vi "PIDDriveLooped.vi"() -> ()   [LabVIEW 2016]
uses:
  <vilib>/Rock Robotics/WPI/Utilities/WPI_GetSetVariantRefNum.vi
  <vilib>/addons/control/pid/pid.llb/PID (DBL).vi
  <vilib>/addons/control/pid/NI_PID_pid.lvlib
panel:
  in  "Finished PID":bool
  in  "Send":bool
  in  "Amount of Time (s)":dbl=7.0 format="%#_13g"
  out "Verify Graph":cluster{"X":dbl, "Y":dbl}[](graph)=[{"X"=0.0, "Y"=0.0}, {"X"=0.002403834311457255, "Y"=0.41939849398766105}, {"X"=0.009592158448876828, "Y"=0.8359196178093844}, {"X"=0.021530204216830304, "Y"=1.24957688435348}, {"X"=0.03818320341988926, "Y"=1.6603838065082581}, {"X"=0.05951638786262529, "Y"=2.0683538971620288}, {"X"=0.08549498934960995, "Y"=2.473500669203102}, {"X"=0.11608423968541483, "Y"=2.8758376355197877}, {"X"=0.15124937067461156, "Y"=3.2753783090003963}, {"X"=0.1909556141217717, "Y"=3.6721362025332374}, {"X"=0.23516820183146672, "Y"=4.066124829006621}, {"X"=0.2838523656082683, "Y"=4.457357701308857}, {"X"=0.3369733372567481, "Y"=4.8458483323282575}, {"X"=0.39449634858147764, "Y"=5.231610234953131}, {"X"=0.45638663138702834, "Y"=5.614656922071786}, {"X"=0.5226094174779721, "Y"=5.995001906572534}, {"X"=0.5931299386588802, "Y"=6.372658701343687}, {"X"=0.6679134267343245, "Y"=6.747640819273552}, {"X"=0.7469251135088762, "Y"=7.11996177325044}, {"X"=0.8301302307871071, "Y"=7.489635076162661}, {"X"=0.917494010373589, "Y"=7.856674240898527}, {"X"=1.0089816840728933, "Y"=8.221092780346344}, {"X"=1.1045584836895912, "Y"=8.582904207394426}, {"X"=1.204189641028255, "Y"=8.942122034931081}, {"X"=1.307840387893456, "Y"=9.298759775844621}, {"X"=1.4154759560897654, "Y"=9.652830943023353}, {"X"=1.5270615774217553, "Y"=10.004349049355591}, {"X"=1.6425624836939967, "Y"=10.35332760772964}, {"X"=1.761943906711062, "Y"=10.699780131033815}, {"X"=1.8851710782775222, "Y"=11.043720132156423}, {"X"=2.012209230197948, "Y"=11.385161123985775}, {"X"=2.1430235942769134, "Y"=11.72411661941018}, {"X"=2.2775794023189886, "Y"=12.060600131317951}, {"X"=2.4158418861287445, "Y"=12.394625172597397}, {"X"=2.5577762775107535, "Y"=12.726205256136824}, {"X"=2.703347808269587, "Y"=13.055353894824547}, {"X"=2.852521710209817, "Y"=13.382084601548875}, {"X"=3.0052632151360132, "Y"=13.706410889198114}, {"X"=3.1615375548527505, "Y"=14.028346270660581}, {"X"=3.3213099611645984, "Y"=14.347904258824581}, {"X"=3.4845456658761282, "Y"=14.665098366578427}, {"X"=3.651209900791912, "Y"=14.979942106810427}, {"X"=3.8212678977165218, "Y"=15.292448992408891}, {"X"=3.994684888454529, "Y"=15.60263253626213}, {"X"=4.171426104810503, "Y"=15.910506251258454}, {"X"=4.351456778589019, "Y"=16.216083650286173}, {"X"=4.534742141594647, "Y"=16.519378246233597}, {"X"=4.721247425631958, "Y"=16.820403551989035}, {"X"=4.910937862505524, "Y"=17.1191730804408}, {"X"=5.103778684019918, "Y"=17.415700344477198}, {"X"=5.29973512197971, "Y"=17.70999885698654}, {"X"=5.49877240818947, "Y"=18.00208213085714}, {"X"=5.700855774453773, "Y"=18.291963678977307}, {"X"=5.905950452577187, "Y"=18.579657014235345}, {"X"=6.114021674364287, "Y"=18.86517564951957}, {"X"=6.325034671619644, "Y"=19.148533097718293}, {"X"=6.538954676147828, "Y"=19.429742871719817}, {"X"=6.755746919753412, "Y"=19.708818484412458}, {"X"=6.975376634240967, "Y"=19.985773448684526}, {"X"=7.197809051415063, "Y"=20.26062127742433}, {"X"=7.423009403080272, "Y"=20.533375483520178}, {"X"=7.650942921041169, "Y"=20.804049579860383}, {"X"=7.881574837102323, "Y"=21.072657079333254}, {"X"=8.114870383068304, "Y"=21.3392114948271}, {"X"=8.350794790743688, "Y"=21.60372633923023}, {"X"=8.589313291933044, "Y"=21.866215125430962}, {"X"=8.830391118440943, "Y"=22.126691366317594}, {"X"=9.073993502071957, "Y"=22.385168574778447}, {"X"=9.320085674630658, "Y"=22.641660263701823}, {"X"=9.568632867921615, "Y"=22.896179945976034}, {"X"=9.819600313749405, "Y"=23.148741134489395}, {"X"=10.072953243918592, "Y"=23.399357342130212}, {"X"=10.328656890233757, "Y"=23.648042081786798}, {"X"=10.586676484499463, "Y"=23.894808866347457}, {"X"=10.846977258520285, "Y"=24.1396712087005}, {"X"=11.109524444100801, "Y"=24.382642621734245}, {"X"=11.37428327304557, "Y"=24.62373661833699}, {"X"=11.641218977159173, "Y"=24.86296671139706}, {"X"=11.910296788246178, "Y"=25.10034641380275}, {"X"=12.181481938111158, "Y"=25.335889238442384}, {"X"=12.454739658558681, "Y"=25.569608698204256}, {"X"=12.73003518139332, "Y"=25.801518305976685}, {"X"=13.007333738419652, "Y"=26.03163157464799}, {"X"=13.28660056144224, "Y"=26.259962017106464}, {"X"=13.567800882265669, "Y"=26.486523146240437}, {"X"=13.850899932694494, "Y"=26.711328474938195}, {"X"=14.135862944533296, "Y"=26.934391516088066}, {"X"=14.422655149586644, "Y"=27.155725782578354}, {"X"=14.71124177965911, "Y"=27.37534478729736}, {"X"=15.001588066555268, "Y"=27.593262043133414}, {"X"=15.293659242079684, "Y"=27.809491062974814}, {"X"=15.587420538036941, "Y"=28.024045359709874}, {"X"=15.882837186231594, "Y"=28.2369384462269}, {"X"=16.179874418468227, "Y"=28.448183835414202}, {"X"=16.478497466551406, "Y"=28.65779504016009}, {"X"=16.778671562285712, "Y"=28.86578557335288}, {"X"=17.0803619374757, "Y"=29.072168947880872}, {"X"=17.383533823925948, "Y"=29.27695867663239}, {"X"=17.68815245344104, "Y"=29.480168272495728}, {"X"=17.994183057825534, "Y"=29.68181124835921}, {"X"=18.301590868884006, "Y"=29.881901117111138}, {"X"=18.610341118421022, "Y"=30.080451391639823}, {"X"=18.920399038241168, "Y"=30.277475584833578}, {"X"=19.231729860149, "Y"=30.472987209580708}, {"X"=19.544298815949094, "Y"=30.666999778769537}, {"X"=19.85807113744602, "Y"=30.85952680528835}, {"X"=20.17301205644436, "Y"=31.050581802025476}, {"X"=20.48908680474868, "Y"=31.240178281869227}, {"X"=20.806260614163545, "Y"=31.4283297577079}, {"X"=21.124498716493537, "Y"=31.615049742429814}, {"X"=21.443766343543214, "Y"=31.80035174892328}, {"X"=21.76402872711716, "Y"=31.9842492900766}, {"X"=22.085251099019942, "Y"=32.16675587877809}, {"X"=22.40739869105613, "Y"=32.34788502791606}, {"X"=22.730436735030306, "Y"=32.52765025037882}, {"X"=23.054330462747025, "Y"=32.70606505905467}, {"X"=23.379045106010867, "Y"=32.88314296683194}, {"X"=23.704545896626406, "Y"=33.05889748659892}, {"X"=24.030798066398216, "Y"=33.23334213124394}, {"X"=24.35776684713085, "Y"=33.4064904136553}, {"X"=24.685417470628895, "Y"=33.578355846721294}, {"X"=25.01371516869693, "Y"=33.74895194333026}, {"X"=25.342625173139517, "Y"=33.918292216370496}, {"X"=25.672112715761223, "Y"=34.086390178730305}, {"X"=26.002143028366618, "Y"=34.253259343298005}, {"X"=26.332681342760296, "Y"=34.418913222961905}, {"X"=26.6636928907468, "Y"=34.58336533061032}, {"X"=26.995142904130716, "Y"=34.746629179131546}, {"X"=27.326996614716613, "Y"=34.908718281413904}, {"X"=27.659219254309065, "Y"=35.06964615034571}, {"X"=27.99177605471265, "Y"=35.229426298815255}, {"X"=28.32463224773192, "Y"=35.388072239710866}, {"X"=28.657753065171462, "Y"=35.54559748592085}, {"X"=28.99110373883584, "Y"=35.702015550333506}, {"X"=29.32464950052963, "Y"=35.857339945837154}, {"X"=29.658355582057403, "Y"=36.0115841853201}, {"X"=29.99218721522374, "Y"=36.16476178167067}, {"X"=30.32610963183319, "Y"=36.31688624777715}, {"X"=30.660088063690345, "Y"=36.46797109652786}, {"X"=30.994087742599767, "Y"=36.61802984081111}, {"X"=31.328073900366025, "Y"=36.76707599351521}, {"X"=31.662011768793697, "Y"=36.915123067528484}, {"X"=31.995866579687355, "Y"=37.06218457573921}, {"X"=32.32960356485157, "Y"=37.20827403103572}, {"X"=32.66318795609092, "Y"=37.353404946306334}, {"X"=32.99658498520996, "Y"=37.497590834439336}, {"X"=33.329759884013264, "Y"=37.64084520832305}, {"X"=33.66267788430541, "Y"=37.78318158084579}, {"X"=33.99530421789097, "Y"=37.92461346489586}, {"X"=34.327604116574534, "Y"=38.06515437336158}, {"X"=34.65954281216064, "Y"=38.20481781913123}, {"X"=34.991085536453866, "Y"=38.34361731509315}, {"X"=35.32219752125879, "Y"=38.481566374135646}, {"X"=35.65284399838, "Y"=38.618678509147024}, {"X"=35.98299019962205, "Y"=38.754967233015584}, {"X"=36.31260135678951, "Y"=38.89044605862966}, {"X"=36.64164270168696, "Y"=39.025128498877535}, {"X"=36.97007946611896, "Y"=39.15902806664754}, {"X"=37.2978768818901, "Y"=39.29215827482796}, {"X"=37.62500018080493, "Y"=39.424532636307134}, {"X"=37.95141459466804, "Y"=39.55616466397336}, {"X"=38.27708535528399, "Y"=39.68706787071495}, {"X"=38.601977694457354, "Y"=39.81725576942021}, {"X"=38.92605684399272, "Y"=39.946741872977455}, {"X"=39.249288035694626, "Y"=40.07553969427498}, {"X"=39.57163650136766, "Y"=40.203662746201125}, {"X"=39.893067472816405, "Y"=40.331124541644165}, {"X"=40.21354618184543, "Y"=40.45793859349244}, {"X"=40.53303786025929, "Y"=40.58411841463423}, {"X"=40.85150773986257, "Y"=40.70967751795787}, {"X"=41.16892105245982, "Y"=40.834629416351675}, {"X"=41.48524302985565, "Y"=40.95898762270393}, {"X"=41.80043890385462, "Y"=41.08276564990297}, {"X"=42.11447390626127, "Y"=41.205977010837074}, {"X"=42.427313268880205, "Y"=41.328635218394574}, {"X"=42.738922223515985, "Y"=41.45075378546379}, {"X"=43.04926600197319, "Y"=41.57234622493301}, {"X"=43.35830983605638, "Y"=41.69342604969056}, {"X"=43.666018957570124, "Y"=41.81400677262473}, {"X"=43.972358598319005, "Y"=41.934101906623845}, {"X"=44.27729399010758, "Y"=42.053724964576226}, {"X"=44.58079036474045, "Y"=42.172889459370154}, {"X"=44.882812954022164, "Y"=42.29160890389396}, {"X"=45.18332698975728, "Y"=42.40989681103595}, {"X"=45.48229770375039, "Y"=42.527766693684434}, {"X"=45.77969032780607, "Y"=42.64523206472772}, {"X"=46.07547009372889, "Y"=42.76230643705412}, {"X"=46.369602233323405, "Y"=42.87900332355195}, {"X"=46.662051978394196, "Y"=42.995336237109505}, {"X"=46.952784560745826, "Y"=43.11131869061511}, {"X"=47.2417652121829, "Y"=43.22696419695706}, {"X"=47.52895916450995, "Y"=43.34228626902369}, {"X"=47.81433164953157, "Y"=43.45729841970327}, {"X"=48.09784789905231, "Y"=43.57201416188414}, {"X"=48.37947314487676, "Y"=43.686447008454614}, {"X"=48.6591726188095, "Y"=43.80061047230299}, {"X"=48.93691155265508, "Y"=43.914518066317584}, {"X"=49.212655178218085, "Y"=44.02818330338668}, {"X"=49.48636872730308, "Y"=44.14161969639863}, {"X"=49.75801743171465, "Y"=44.25484075824171}, {"X"=50.027566523257335, "Y"=44.36786000180426}, {"X"=50.29498123373574, "Y"=44.48069093997457}, {"X"=50.56022679495441, "Y"=44.59334708564095}, {"X"=50.823268438717946, "Y"=44.70584195169171}, {"X"=51.08407139683091, "Y"=44.818189051015175}, {"X"=51.34260090109785, "Y"=44.93040189649964}, {"X"=51.59882218332336, "Y"=45.04249400103342}, {"X"=51.852700475312005, "Y"=45.154478877504815}, {"X"=52.10420100886837, "Y"=45.26637003880216}, {"X"=52.353289015797, "Y"=45.378180997813736}, {"X"=52.59992972790249, "Y"=45.48992526742788}, {"X"=52.8440883769894, "Y"=45.60161636053288}, {"X"=53.08573019486229, "Y"=45.713267790017056}, {"X"=53.32482041332578, "Y"=45.824893068768716}, {"X"=53.561324264184385, "Y"=45.93650570967617}, {"X"=53.7952069792427, "Y"=46.04811922562773}, {"X"=54.0264337903053, "Y"=46.159747129511715}, {"X"=54.25496992917675, "Y"=46.27140293421641}, {"X"=54.48078062766162, "Y"=46.38310015263014}, {"X"=54.7038311175645, "Y"=46.49485229764122}, {"X"=54.92408663068993, "Y"=46.606672882137964}, {"X"=55.14151239884251, "Y"=46.71857541900866}, {"X"=55.356073653826805, "Y"=46.830573421141644}, {"X"=55.56773562744737, "Y"=46.9426804014252}, {"X"=55.77646355150879, "Y"=47.05490987274766}, {"X"=55.98222265781563, "Y"=47.167275347997325}, {"X"=56.18497817817248, "Y"=47.279790340062505}, {"X"=56.3846953443839, "Y"=47.39246836183151}, {"X"=56.58133938825444, "Y"=47.50532292619265}, {"X"=56.77487554158871, "Y"=47.61836754603424}, {"X"=56.96526903619125, "Y"=47.731615734244585}, {"X"=57.15248510386666, "Y"=47.845081003712}, {"X"=57.33648897641948, "Y"=47.95877686732478}, {"X"=57.51724588565432, "Y"=48.07271683797124}, {"X"=57.69472106337571, "Y"=48.186914428539716}, {"X"=57.868879741388234, "Y"=48.30138315191849}, {"X"=58.03968715149649, "Y"=48.416136520995884}, {"X"=58.20710852550503, "Y"=48.5311880486602}, {"X"=58.37110909521841, "Y"=48.64655124779974}, {"X"=58.53165409244122, "Y"=48.76223963130285}, {"X"=58.68870874897804, "Y"=48.8782667120578}, {"X"=58.84223829663342, "Y"=48.994646002952926}, {"X"=58.99220796721195, "Y"=49.11139101687652}, {"X"=59.138582992518195, "Y"=49.2285152667169}, {"X"=59.28132860435671, "Y"=49.34603226536239}, {"X"=59.4204100345321, "Y"=49.46395552570128}, {"X"=59.55579251484891, "Y"=49.58229856062189}, {"X"=59.68744127711172, "Y"=49.70107488301252}, {"X"=59.8153215531251, "Y"=49.82029800576148}, {"X"=59.93939857469362, "Y"=49.9399814417571}, {"X"=60.05963857964622, "Y"=50.060138261910026}, {"X"=60.176030944371796, "Y"=50.18077137164493}, {"X"=60.2885881838193, "Y"=50.30187351090052}, {"X"=60.397323818962015, "Y"=50.42343697763785}, {"X"=60.50225137077323, "Y"=50.545454069817964}, {"X"=60.60338436022622, "Y"=50.6679170854019}, {"X"=60.70073630829428, "Y"=50.790818322350724}, {"X"=60.794320735950684, "Y"=50.914150078625475}, {"X"=60.88415116416872, "Y"=51.03790465218721}, {"X"=60.97024111392168, "Y"=51.16207434099697}, {"X"=61.052604106182834, "Y"=51.286651443015806}, {"X"=61.13125366192548, "Y"=51.411628256204764}, {"X"=61.20620330212289, "Y"=51.5369970785249}, {"X"=61.27746654774836, "Y"=51.66275020793726}, {"X"=61.34505691977516, "Y"=51.788879942402886}, {"X"=61.40898793917659, "Y"=51.91537857988284}, {"X"=61.46927312692593, "Y"=52.04223841833816}, {"X"=61.52592600399646, "Y"=52.169451755729895}, {"X"=61.578960091361466, "Y"=52.2970108900191}, {"X"=61.628388909994236, "Y"=52.42490811916683}, {"X"=61.674225980868044, "Y"=52.55313574113411}, {"X"=61.71648482495618, "Y"=52.68168605388202}, {"X"=61.75517896323194, "Y"=52.81055135537158}, {"X"=61.79032191666859, "Y"=52.93972394356386}, {"X"=61.82192720623943, "Y"=53.069196116419896}, {"X"=61.850008352917726, "Y"=53.198960171900744}, {"X"=61.87457887767678, "Y"=53.32900840796744}, {"X"=61.89565230148987, "Y"=53.459333122581064}, {"X"=61.91324214533027, "Y"=53.58992661370263}, {"X"=61.92736193017129, "Y"=53.720781179293205}, {"X"=61.93802517698619, "Y"=53.85188911731383}, {"X"=61.945245406748256, "Y"=53.98324272572556}, {"X"=61.94903614043079, "Y"=54.11483430248945}, {"X"=61.94941089900706, "Y"=54.24665614556653}, {"X"=61.94638320345036, "Y"=54.37870055291786}, {"X"=61.939966574733965, "Y"=54.51095982250449}, {"X"=61.93017453383116, "Y"=54.64342625228747}, {"X"=61.917020601715244, "Y"=54.776092140227846}, {"X"=61.90051829935948, "Y"=54.90894978428667}, {"X"=61.88068114773718, "Y"=55.041991482424976}, {"X"=61.8575226678216, "Y"=55.17520953260384}, {"X"=61.831056380586034, "Y"=55.30859623278428}, {"X"=61.801295807003775, "Y"=55.44214388092737}, {"X"=61.7682544680481, "Y"=55.57584477499415}, {"X"=61.73194588469229, "Y"=55.709691212945664}, {"X"=61.69238357790963, "Y"=55.84367549274297}, {"X"=61.64958106867341, "Y"=55.977789912347106}, {"X"=61.60355187795692, "Y"=56.11202676971913}, {"X"=61.554309526733434, "Y"=56.24637836282009}, {"X"=61.50186753597624, "Y"=56.380836989611026}, {"X"=61.446239426658614, "Y"=56.515394948053}, {"X"=61.38743871975385, "Y"=56.650044536107046}, {"X"=61.32547893623523, "Y"=56.784778051734236}, {"X"=61.26037359707603, "Y"=56.9195877928956}, {"X"=61.192136223249555, "Y"=57.054466057552176}, {"X"=61.12078033572907, "Y"=57.18940514366504}, {"X"=61.046319455487875, "Y"=57.32439734919522}, {"X"=60.96876710349924, "Y"=57.459434972103786}, {"X"=60.88813680073645, "Y"=57.59451031035177}, {"X"=60.8044420681728, "Y"=57.729615661900226}, {"X"=60.717696426781565, "Y"=57.864743324710204}, {"X"=60.627913397536034, "Y"=57.99988559674275}, {"X"=60.53510650140949, "Y"=58.13503477595891}, {"X"=60.439289259375215, "Y"=58.27018316031974}, {"X"=60.3404751924065, "Y"=58.40532304778628}, {"X"=60.23867782147662, "Y"=58.540446736319595}, {"X"=60.133910667558865, "Y"=58.67554652388072}, {"X"=60.026187251626524, "Y"=58.8106147084307}, {"X"=59.915521094652874, "Y"=58.9456435879306}, {"X"=59.801925717611205, "Y"=59.08062546034145}, {"X"=59.68541464147479, "Y"=59.21555262362432}, {"X"=59.56600138721692, "Y"=59.35041737574024}, {"X"=59.443699475810895, "Y"=59.48521201465027}, {"X"=59.31852242822997, "Y"=59.61992883831546}, {"X"=59.19048376544745, "Y"=59.754560144696846}, {"X"=59.05959700843661, "Y"=59.8890982317555}, {"X"=58.92587567817074, "Y"=60.02353539745244}, {"X"=58.78933329562313, "Y"=60.15786393974874}, {"X"=58.64998338176704, "Y"=60.29207615660544}, {"X"=58.50783945757579, "Y"=60.42616434598358}, {"X"=58.36291504402263, "Y"=60.56012080584423}, {"X"=58.21522366208086, "Y"=60.69393783414842}, {"X"=58.064778832723775, "Y"=60.8276077288572}, {"X"=57.91159407692464, "Y"=60.96112278793164}, {"X"=57.75568291565674, "Y"=61.094475309332765}, {"X"=57.59705886989338, "Y"=61.227657591021625}, {"X"=57.43573546060783, "Y"=61.36066193095929}, {"X"=57.27172620877337, "Y"=61.493480627106784}, {"X"=57.10504463536329, "Y"=61.62610597742517}, {"X"=56.93570426135088, "Y"=61.7585302798755}, {"X"=56.763718607709414, "Y"=61.89074583241881}, {"X"=56.58910119541218, "Y"=62.022744933016156}, {"X"=56.41186554543247, "Y"=62.15451987962858}, {"X"=56.23202517874355, "Y"=62.28606297021715}, {"X"=56.04959361631872, "Y"=62.4173665027429}, {"X"=55.86458437913127, "Y"=62.54842277516687}, {"X"=55.67701098815446, "Y"=62.67922408545013}, {"X"=55.4868869643616, "Y"=62.80976273155371}, {"X"=55.294225828725956, "Y"=62.94003101143868}, {"X"=55.099041102220816, "Y"=63.07002122306607}, {"X"=54.90134630581948, "Y"=63.19972566439694}, {"X"=54.70115496049521, "Y"=63.329136633392324}, {"X"=54.498480587221316, "Y"=63.45824642801328}, {"X"=54.29333670697105, "Y"=63.58704734622087}, {"X"=54.085736840717715, "Y"=63.71553168597613}, {"X"=53.8756945094346, "Y"=63.8436917452401}, {"X"=53.66322323409498, "Y"=63.97151982197384}, {"X"=53.448336535672134, "Y"=64.09900821413841}, {"X"=53.23104793513937, "Y"=64.22614921969483}, {"X"=53.01137095346995, "Y"=64.35293513660417}, {"X"=52.78931911163717, "Y"=64.47935826282747}, {"X"=52.564905930614295, "Y"=64.60541089632581}, {"X"=52.33814493137463, "Y"=64.73108533506019}, {"X"=52.10904963489146, "Y"=64.85637387699168}, {"X"=51.87763356213806, "Y"=64.98126882008134}, {"X"=51.64391023408773, "Y"=65.10576246229019}, {"X"=51.40789317171371, "Y"=65.22984710157931}, {"X"=51.16959589598933, "Y"=65.35351503590974}, {"X"=50.92903192788787, "Y"=65.47675856324251}, {"X"=50.68621478838259, "Y"=65.59956998153869}, {"X"=50.44115799844681, "Y"=65.72194158875934}, {"X"=50.19387507905377, "Y"=65.84386568286547}, {"X"=49.94437955117677, "Y"=65.96533456181817}, {"X"=49.69268493578913, "Y"=66.08634052357844}, {"X"=49.43880475386409, "Y"=66.2068758661074}, {"X"=49.18275252637494, "Y"=66.32693288736603}, {"X"=48.924541774295, "Y"=66.4465038853154}, {"X"=48.66418601859751, "Y"=66.56558115791657}, {"X"=48.40169878025579, "Y"=66.6841570031306}, {"X"=48.13709358024309, "Y"=66.8022237189185}, {"X"=47.870383939532715, "Y"=66.91977360324137}, {"X"=47.60158337909796, "Y"=67.0367989540602}, {"X"=47.33070541991208, "Y"=67.15329206933609}, {"X"=47.05776358294839, "Y"=67.26924524703006}, {"X"=46.78277138918015, "Y"=67.38465078510316}, {"X"=46.50574235958064, "Y"=67.49950098151646}, {"X"=46.22669001512318, "Y"=67.61378813423099}, {"X"=45.94562787678102, "Y"=67.72750454120781}, {"X"=45.66256946552747, "Y"=67.84064250040795}, {"X"=45.37752830233579, "Y"=67.95319430979248}, {"X"=45.090517908179265, "Y"=68.06515226732245}, {"X"=44.80155180403122, "Y"=68.17650867095887}, {"X"=44.51064351086487, "Y"=68.28725581866284}, {"X"=44.217806549653574, "Y"=68.39738600839539}, {"X"=43.92305444137057, "Y"=68.50689153811756}, {"X"=43.62640070698913, "Y"=68.6157647057904}, {"X"=43.32785886748259, "Y"=68.72399780937496}, {"X"=43.027442443824185, "Y"=68.83158314683232}, {"X"=42.72516495698723, "Y"=68.93851301612347}, {"X"=42.42103992794502, "Y"=69.0447797152095}, {"X"=42.11508087767078, "Y"=69.15037554205145}, {"X"=41.807301327137864, "Y"=69.25529279461037}, {"X"=41.4977147973195, "Y"=69.3595237708473}, {"X"=41.186334809189006, "Y"=69.46306076872331}, {"X"=40.87317488371967, "Y"=69.56589608619943}, {"X"=40.558248541884744, "Y"=69.66802202123671}, {"X"=40.24156930465756, "Y"=69.7694308717962}, {"X"=39.92315069301135, "Y"=69.87011493583896}, {"X"=39.60300622791944, "Y"=69.97006651132602}, {"X"=39.28114943035509, "Y"=70.06927789621844}, {"X"=38.95759382129158, "Y"=70.16774138847728}, {"X"=38.632352921702235, "Y"=70.26544928606356}, {"X"=38.30544025256029, "Y"=70.36239388693835}, {"X"=37.97686933483905, "Y"=70.4585674890627}, {"X"=37.646653689511815, "Y"=70.55396239039766}, {"X"=37.31480683755183, "Y"=70.64857088890426}, {"X"=36.98134229993241, "Y"=70.74238528254357}, {"X"=36.646273597626845, "Y"=70.83539786927662}, {"X"=36.309614251608394, "Y"=70.92760094706448}, {"X"=35.971377782850375, "Y"=71.01898681386817}, {"X"=35.63157771232602, "Y"=71.10954776764878}, {"X"=35.290227561008656, "Y"=71.19927610636732}, {"X"=34.94734084987158, "Y"=71.28816412798486}, {"X"=34.602931099888025, "Y"=71.37620413046244}, {"X"=34.257011832031324, "Y"=71.46338841176112}, {"X"=33.909596567274704, "Y"=71.54970926984194}, {"X"=33.560698826591505, "Y"=71.63515900266594}, {"X"=33.21033213095501, "Y"=71.71972990819418}, {"X"=32.85851000133846, "Y"=71.80341428438771}, {"X"=32.50524595871519, "Y"=71.8862044292076}, {"X"=32.150553524058424, "Y"=71.96809264061484}, {"X"=31.794446218341495, "Y"=72.04907121657052}, {"X"=31.436937562537693, "Y"=72.1291324550357}, {"X"=31.07804107762026, "Y"=72.2082686539714}, {"X"=30.717770284562526, "Y"=72.2864721113387}, {"X"=30.356138704337727, "Y"=72.36373512509861}, {"X"=29.99315985791917, "Y"=72.4400499932122}, {"X"=29.628847266280175, "Y"=72.51540901364052}, {"X"=29.26321445039396, "Y"=72.58980448434463}, {"X"=28.896274931233847, "Y"=72.66322870328555}, {"X"=28.528042229773142, "Y"=72.73567396842435}, {"X"=28.158529866985077, "Y"=72.80713257772207}, {"X"=27.787751363842986, "Y"=72.87759682913976}, {"X"=27.41572024132011, "Y"=72.94705902063848}, {"X"=27.042450020389744, "Y"=73.01551145017926}, {"X"=26.66795422202521, "Y"=73.08294641572316}, {"X"=26.292246367199745, "Y"=73.14935621523124}, {"X"=25.915339976886678, "Y"=73.21473314666451}, {"X"=25.537248572059234, "Y"=73.27906950798408}, {"X"=25.15798567369074, "Y"=73.34235759715094}, {"X"=24.77756480275449, "Y"=73.40458971212617}, {"X"=24.395999480223722, "Y"=73.46575815087081}, {"X"=24.01330322707178, "Y"=73.52585521134591}, {"X"=23.629489564271893, "Y"=73.58487319151253}, {"X"=23.244572012797356, "Y"=73.6428043893317}, {"X"=22.85856409362151, "Y"=73.69964110276447}, {"X"=22.471479327717553, "Y"=73.7553756297719}, {"X"=22.083331236058854, "Y"=73.81000026831504}, {"X"=21.694133339618624, "Y"=73.86350731635494}, {"X"=21.30389915937016, "Y"=73.91588907185263}, {"X"=20.912642216286805, "Y"=73.96713783276918}, {"X"=20.520376031341776, "Y"=74.01724589706564}, {"X"=20.127114125508392, "Y"=74.06620556270303}, {"X"=19.732870019759957, "Y"=74.11400912764242}, {"X"=19.337657235069685, "Y"=74.16064888984488}, {"X"=18.941489292410935, "Y"=74.20611714727141}, {"X"=18.544379712756943, "Y"=74.2504061978831}, {"X"=18.146342017081004, "Y"=74.29350833964098}, {"X"=17.747389726356438, "Y"=74.3354158705061}, {"X"=17.34753636155647, "Y"=74.3761210884395}, {"X"=16.946795443654445, "Y"=74.41561629140226}, {"X"=16.545180493623583, "Y"=74.4538937773554}, {"X"=16.142705032437206, "Y"=74.49094584425998}, {"X"=15.739382581068632, "Y"=74.52676479007707}, {"X"=15.33522666049106, "Y"=74.56134291276766}, {"X"=14.93025079167785, "Y"=74.59467251029285}, {"X"=14.524468495602243, "Y"=74.62674588061368}, {"X"=14.117893293237543, "Y"=74.65755532169119}, {"X"=13.710538705557042, "Y"=74.68709313148642}, {"X"=13.302418253533986, "Y"=74.71535160796044}, {"X"=12.893545458141716, "Y"=74.74232304907429}, {"X"=12.483933840353458, "Y"=74.76799975278902}, {"X"=12.073596921142531, "Y"=74.79237401706567}, {"X"=11.662548221482247, "Y"=74.81543813986531}, {"X"=11.250801262345803, "Y"=74.83718441914895}, {"X"=10.83836956470656, "Y"=74.85760515287768}, {"X"=10.425266649537782, "Y"=74.87669263901253}, {"X"=10.011506037812751, "Y"=74.89443917551456}, {"X"=9.597101250504764, "Y"=74.9108370603448}, {"X"=9.182065808587055, "Y"=74.92587859146431}, {"X"=8.766413233032956, "Y"=74.93955606683414}, {"X"=8.35015704481576, "Y"=74.95186178441534}, {"X"=7.933310764908711, "Y"=74.96278804216897}, {"X"=7.515887914285145, "Y"=74.97232713805604}, {"X"=7.097902013918272, "Y"=74.98047137003763}, {"X"=6.679366584781441, "Y"=74.98721303607478}, {"X"=6.260295147847927, "Y"=74.99254443412855}, {"X"=5.840701224090978, "Y"=74.99645786215997}, {"X"=5.420598334483934, "Y"=74.99894561813011}, {"X"=5.000000000000007, "Y"=75.0}]
  in  "PID Segments (1-500)":dbl=150.0
  in  "Limit of Orientation Change":dbl=30.0
  in  "Absolute Theta Final":dbl=-1.57
  in  "Absolute Theta initial":dbl
  in  "Y":dbl[](array[numeric])=[0.0, 60.0, 5.0]
  in  "X":dbl[](array[numeric])=[0.0, 50.0, 75.0]
  out "throttle":dbl=-0.8 format="%.2f"
  out "steer":dbl=0.8 format="%.2f"
  out "Waveform Chart":cluster{dbl, "setpoint":dbl}(graph)={92.439765, "setpoint"=131.40149028791936}
  out "Waveform Chart 2":cluster{"Yaw Wind":dbl, "setpoint":dbl}(graph)={"Yaw Wind"=0.830122225479803, "setpoint"=1.5429574932445604}
  in  "Manual":bool
  in  "Steer Range":cluster{"output high":dbl, "output low":dbl}={"output high"=0.8, "output low"=-0.8} {"output low" format="%.2f"; "output high" format="%.2f"}
  in  "PID Steer gains":T1={"proportional gain (Kc)"=1.0, "integral time (Ti, min)"=0.01, "derivative time (Td, min)"=0.0} {"derivative time (Td, min)" format="%.3f"; "integral time (Ti, min)" format="%.3f"; "proportional gain (Kc)" format="%.3f"}
  in  "Speed Range":cluster{"output high":dbl, "output low":dbl}={"output high"=0.8, "output low"=-0.8} {"output low" format="%.2f"; "output high" format="%.2f"}
  in  "PID Speed gains":T1={"proportional gain (Kc)"=0.04, "integral time (Ti, min)"=0.0, "derivative time (Td, min)"=0.0} {"derivative time (Td, min)" format="%.3f"; "integral time (Ti, min)" format="%.3f"; "proportional gain (Kc)" format="%.3f"}
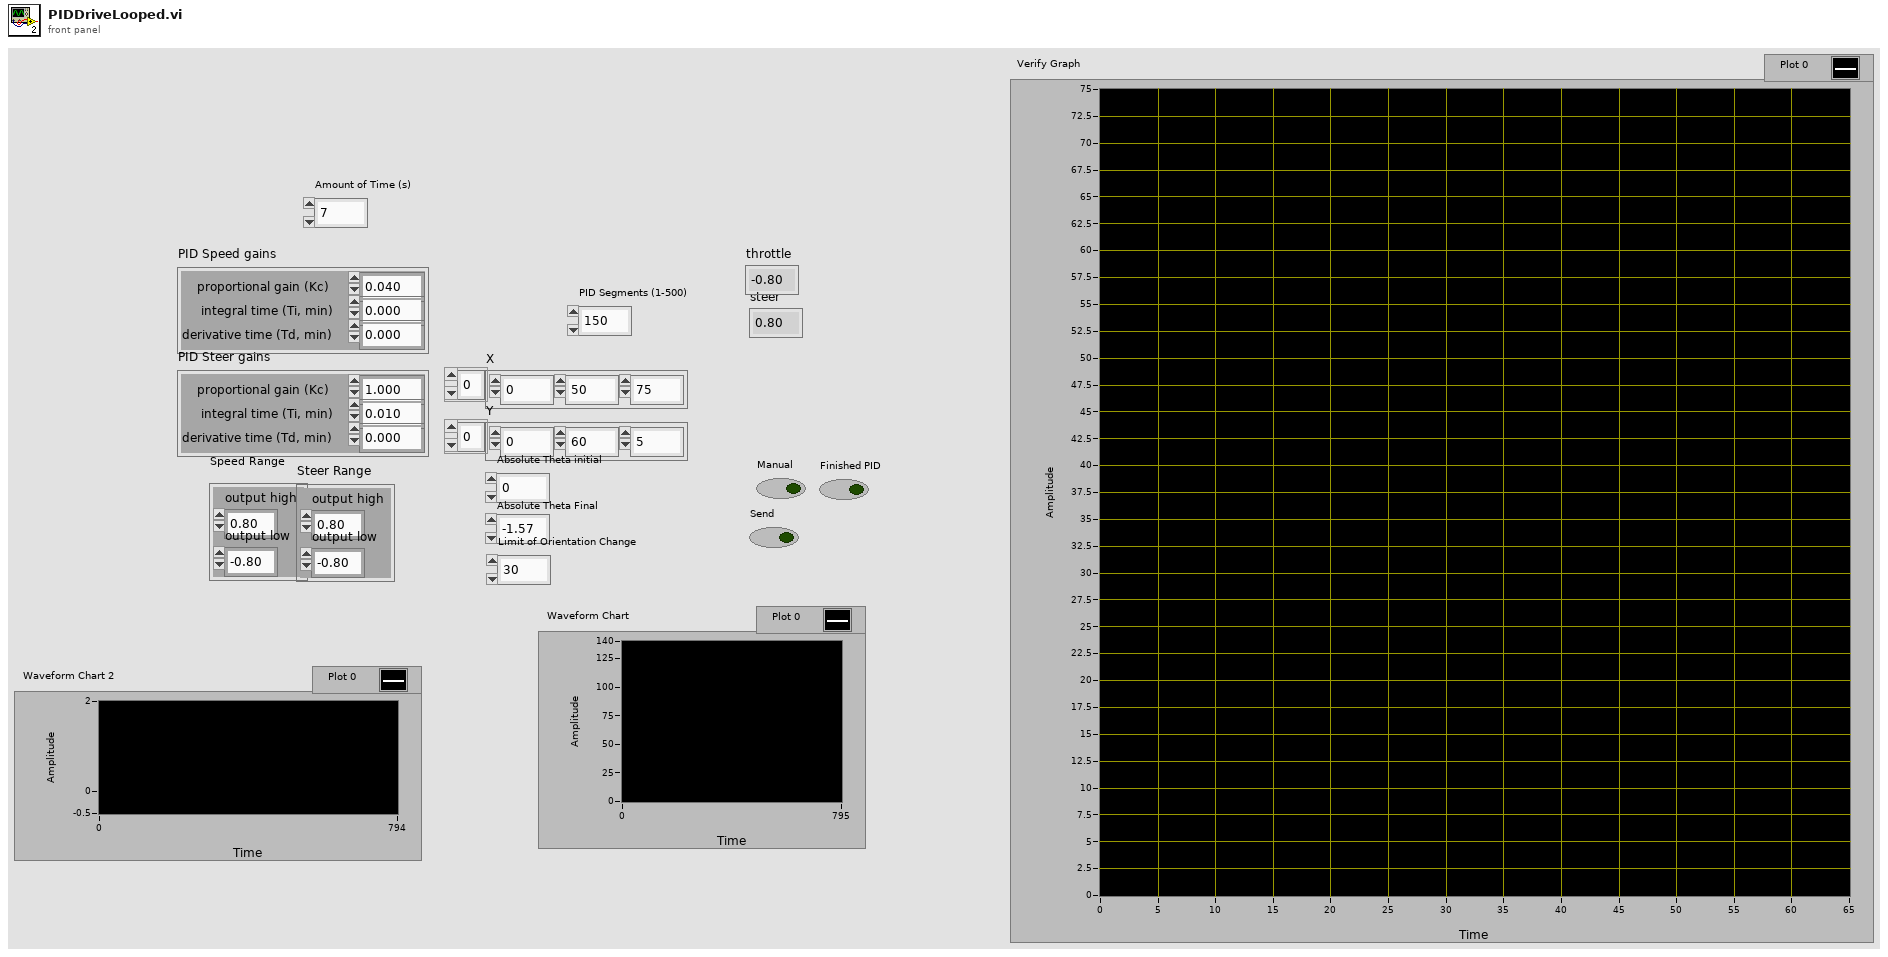
[diagram p1: front panel]
types:
  T1 = cluster{"proportional gain (Kc)":dbl, "integral time (Ti, min)":dbl, "derivative time (Td, min)":dbl}
  T2 = typedef "WPI_MotorControlDeviceRef.ctl" = cluster{"DeviceStatus":errorcluster, "Type":T3, "PWM":cluster{"PWM Channel":T4, "DeadBand":T5}, "CAN":cluster{"Device Number":u8, "SetOutput VI Ref":variant, "GetOutput VI Ref":variant, "Enable VI Ref":variant, "Disable VI Ref":variant, "Data":variant}, "Invert":bool}
  T3 = typedef "WPI_MotorControlType.ctl" = enum16{"PWM", "CAN"}
  T4 = typedef "FPGA_DIOPWMChannel.ctl" = enum8{"PWM 0", "PWM 1", "PWM 2", "PWM 3", "PWM 4", "PWM 5", "PWM 6", "PWM 7", "PWM 8", "PWM 9", "PWM MXP 0", "PWM MXP 1", "PWM MXP 2", "PWM MXP 3", "PWM MXP 4", "PWM MXP 5", "PWM MXP 6", "PWM MXP 7", "PWM MXP 8", "PWM MXP 9", "Invalid"}
  T5 = typedef "WPI_PWMDeadband.ctl" = cluster{"Name":string, "maxPositivePwm":i32, "minPositivePwm":i32, "centerPwm":i32, "maxNegativePwm":i32, "minNegativePwm":i32, "angularRange":u16}
  T6 = typedef "WPI_JoystickDevRef.ctl" = cluster{"Device":T7}
  T7 = typedef "WPI_JoystickDeviceEnum.ctl" = enum16{"USB 0", "USB 1", "USB 2", "USB 3", "USB 4", "USB 5"}
  T8 = typedef "WPI_EncoderDevRef.ctl" = cluster{"DevStatus":errorcluster, "EncoderIndex":T9, "CounterIndex":T10, "DistancePerCount":dbl, "Decoding Type":T11}
  T9 = typedef "FPGA_EncoderIdx.ctl" = enum8{"Enc 0", "Enc 1", "Enc 2", "Enc 3", "Enc 4", "Enc 5", "Enc 6", "Enc 7", "Invalid"}
  T10 = typedef "FPGA_CounterCtrSystemIndex.ctl" = enum8{"Ctr 0", "Ctr 1", "Ctr 2", "Ctr 3", "Ctr 4", "Ctr 5", "Ctr 6", "Ctr 7", "Invalid"}
  T11 = typedef "WPI_EncoderType.ctl" = enum16{"1x", "2x", "4x"}
  T12 = typedef "WPI_I2CDevRef.ctl" = cluster{"DevStatus":errorcluster, "Device Address":u8, "Handle":i32, "I2C Bus":T13}
  T13 = typedef "i2c_bus.ctl" = enum16{"I2C On-Board", "I2C MXP", "Invalid"}
  T14 = cluster{"Yaw":dbl, "Roll":dbl, "Pitch":dbl, "Yaw Wind":dbl, "Roll Wind":dbl, "Pitch Wind":dbl}
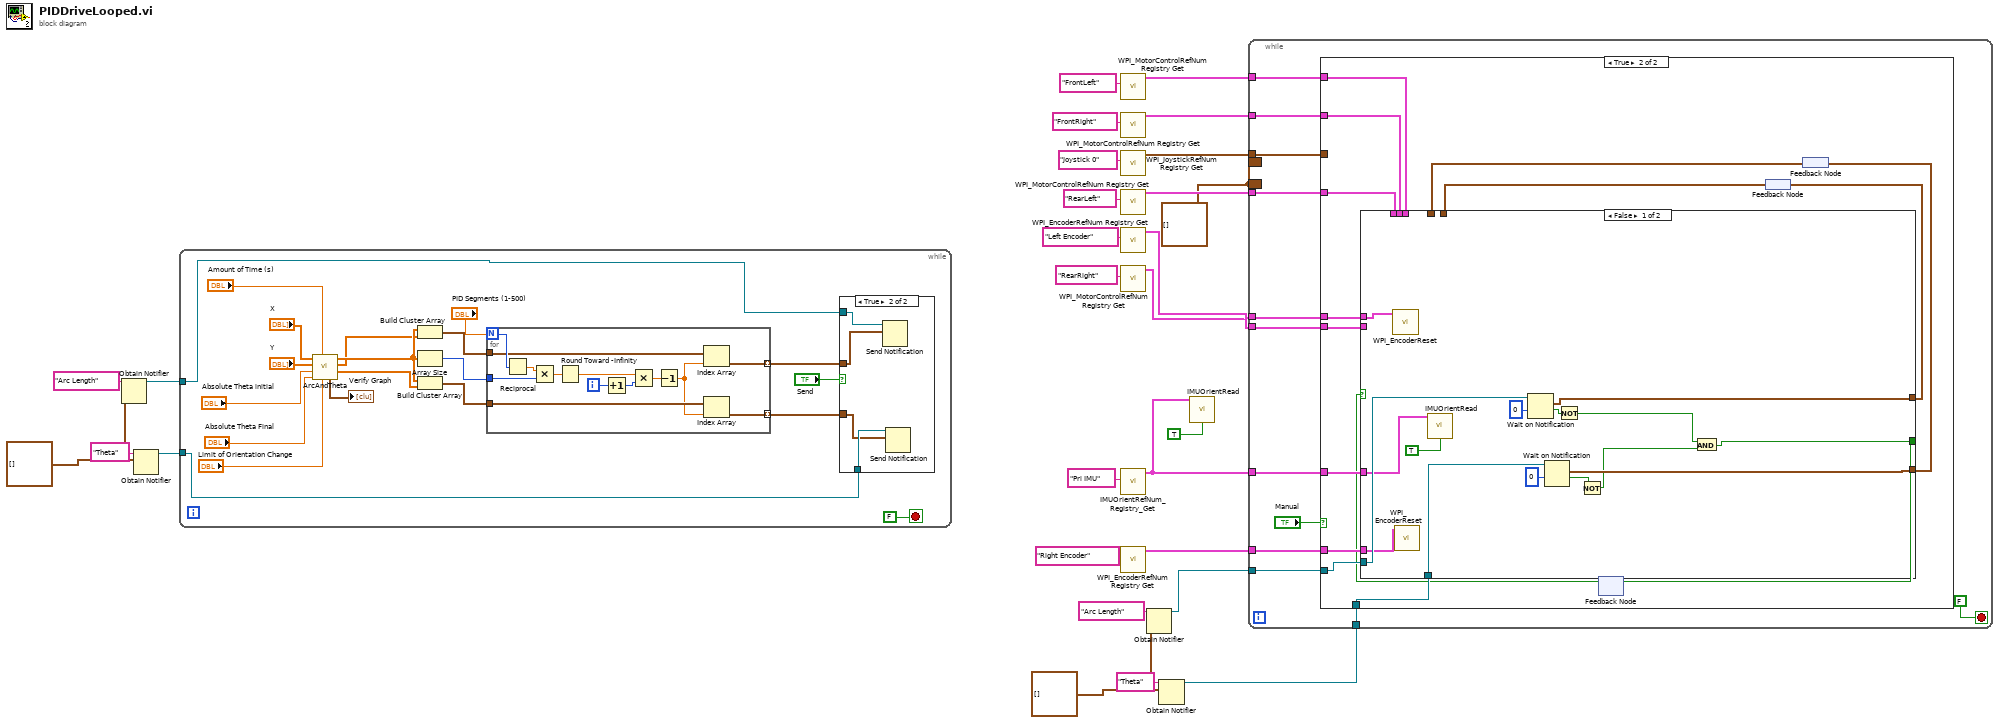
[diagram p0: block diagram]
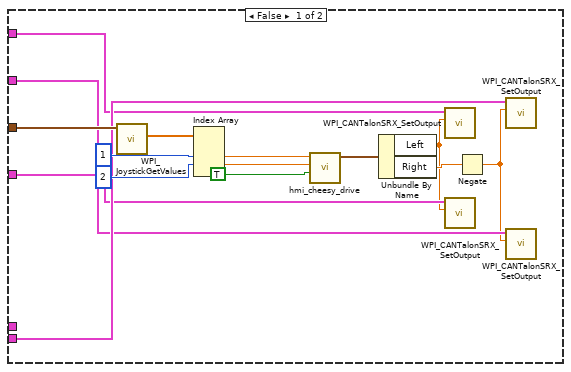
[diagram p3: hidden frame]
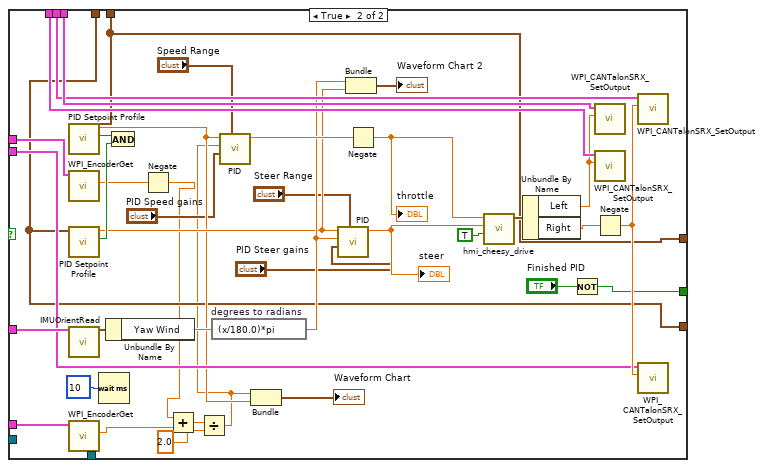
[diagram p4: hidden frame]
diagram:
  w1 = cluster{dbl, dbl}[] [] ("array of clusters")
  w6 = cluster{dbl, dbl}[] [] ("array of clusters")
  w8 = cluster{dbl, dbl}[] [] ("array of clusters")
  n1 = Obtain Notifier(name (unnamed)="Arc Length", notification data type=w8) -> (notifier out=w7:refnum<notifier>)  [unwired: 2 in, 2 out]
  n2 = Obtain Notifier(name (unnamed)="Theta", notification data type=w8) -> (notifier out=w9:refnum<notifier>)  [unwired: 2 in, 2 out]
  n3 = while {
    tunnel: w9 -> [w31]
    tunnel: w7 -> [w30]
    stop <- FALSE stop-if-true
    n4 = call "ArcAndTheta.vi"("Limit of Orientation Change"="Limit of Orientation Change", "Amount of Time (s)"="Amount of Time (s)", "Absolute Theta Final"="Absolute Theta Final", "Absolute Theta initial"="Absolute Theta initial", "Y"="Y", "X"="X") -> ("Theta(arc length)"=w35:dbl[], "Arc Length"=w34:dbl[], "TimeStamp"=w42:dbl[], "Verify Graph"=→"Verify Graph":cluster{"X":dbl, "Y":dbl}[])  [unwired: 2 in]
    n5 = Build Cluster Array(w42, w34) -> (w44:cluster{dbl, dbl}[])
    n6 = Array Size(array=w42) -> (size(s)=w43:i32)
    n7 = Build Cluster Array(w42, w35) -> (w45:cluster{dbl, dbl}[])
    n8 = for {
      N: "PID Segments (1-500)" -> [w65]
      tunnel: w43 -> [w63]
      tunnel: w44 -> [w57]
      tunnel: w45 -> [w56]
      tunnel: [w54] -> w33 mode=indexing
      tunnel: [w53] -> w32 mode=indexing
      i -> [w61]
      n9 = Reciprocal(x=w65) -> (1/x=w64:dbl)
      n10 = Multiply(x=w64, y=w63) -> (x*y=w62:dbl)
      n11 = Round Toward -Infinity(1:w62) -> (0:w59:dbl)
      n12 = Increment(x=w61) -> (x+1=w60:i32)
      n13 = Multiply(x=w59, y=w60) -> (x*y=w58:dbl)
      n14 = Decrement(x=w58) -> (x-1=w55:dbl)
      n15 = Index Array(array=w57, index=w55) -> (element=w54:cluster{dbl, dbl})
      n16 = Index Array(array=w56, index=w55) -> (element=w53:cluster{dbl, dbl})
    }
    n17 = case shown="True" "Send" {
      tunnel: w33 -> [_ w51]
      tunnel: w32 -> [_ w49]
      tunnel: w31 -> [_ w50]
      tunnel: w30 -> [_ w52]
      frame False {
      }
      frame True {
        n18 = Send Notification(notification=w51, notifier=w52) -> ()  [unwired: 1 in, 2 out]
        n19 = Send Notification(notification=w49, notifier=w50) -> ()  [unwired: 1 in, 2 out]
      }
    }
  }
  n20 = call <vilib>:"WPI_MotorControlRefNum Registry Get.vi"("refnum name"="FrontLeft") -> ("MotorControlDevRef"=w15:T2)  [unwired: 9 in, 1 out]
  n21 = call <vilib>:"WPI_MotorControlRefNum Registry Get.vi"("refnum name"="FrontRight") -> ("MotorControlDevRef"=w14:T2)  [unwired: 9 in, 1 out]
  n22 = call <vilib>:"WPI_JoystickRefNum Registry Get.vi"("refnum name"="Joystick 0") -> ("JoystickDevRef"=w20:T6)  [unwired: 9 in, 1 out]
  n23 = call <vilib>:"WPI_MotorControlRefNum Registry Get.vi"("refnum name"="RearLeft") -> ("MotorControlDevRef"=w12:T2)  [unwired: 9 in, 1 out]
  n24 = call <vilib>:"WPI_EncoderRefNum Registry Get.vi"("refnum name"="Left Encoder") -> ("EncoderDevRef"=w26:T8)  [unwired: 9 in, 1 out]
  n25 = call <vilib>:"WPI_MotorControlRefNum Registry Get.vi"("refnum name"="RearRight") -> ("MotorControlDevRef"=w13:T2)  [unwired: 9 in, 1 out]
  n26 = call <userlib>:"IMUOrientRefNum_Registry_Get.vi"("refnum name"="Pri IMU") -> ("I2CDevRef out"=w23:T12)  [unwired: 9 in, 1 out]
  n27 = call <vilib>:"WPI_EncoderRefNum Registry Get.vi"("refnum name"="Right Encoder") -> ("EncoderDevRef"=w27:T8)  [unwired: 9 in, 1 out]
  n28 = Obtain Notifier(name (unnamed)="Arc Length", notification data type=w6) -> (notifier out=w3:refnum<notifier>)  [unwired: 2 in, 2 out]
  n29 = Obtain Notifier(name (unnamed)="Theta", notification data type=w6) -> (notifier out=w2:refnum<notifier>)  [unwired: 2 in, 2 out]
  n30 = call <userlib>:"IMUOrientRead.vi"("I2CDevRef"=w23, "Gyro Reset"=TRUE) -> ()  [unwired: 7 in, 7 out]
  n31 = while {
    tunnel: w27 -> [w76]
    tunnel: w26 -> [w77]
    tunnel: w23 -> [w75]
    tunnel: w20 -> [w72]
    tunnel: w15 -> [w71]
    tunnel: w14 -> [w70]
    tunnel: w13 -> [w69]
    tunnel: w12 -> [w68]
    tunnel: w3 -> [w67]
    tunnel: w2 -> [w66]
    border: w1 -> [_]
    border: w1 -> [_]
    stop <- FALSE stop-if-true
    n32 = case shown="True" "Manual" {
      tunnel: w77 -> [_ w107]
      tunnel: w76 -> [_ w101]
      tunnel: w75 -> [_ w106]
      tunnel: w72 -> [w91 _]
      tunnel: w71 -> [w82 w105]
      tunnel: w70 -> [w84 w103]
      tunnel: w69 -> [w85 w102]
      tunnel: w68 -> [w81 w104]
      tunnel: w67 -> [_ w99]
      tunnel: w66 -> [_ w100]
      frame False {
        n33 = call <vilib>:"WPI_JoystickGetValues.vi"("JoystickDevRef"=w91) -> ("Axes"=w90:dbl[])  [unwired: 6 in, 4 out]
        n34 = Index Array(array=w90, index #2=1 ("index"), index #3=2 ("index")) -> (element #2=w89:dbl, element #3=w88:dbl)  [unwired: 2 in, 2 out]
        n35 = call <userlib>:"hmi_cheesy_drive.vi"("Quick Turn"=TRUE, "Wheel"=w88, "Throttle"=w89) -> ("Drive Data"=w92:cluster{"Left":dbl, "Right":dbl})  [unwired: 8 in]
        n36 = Unbundle By Name(w92) -> ("Left"=w80:dbl, "Right"=w83:dbl)
        n37 = call <vilib>:"WPI_CANTalonSRX_SetOutput.vi"("Output"=w80, "MotorControlDevRef"=w82) -> ()  [unwired: 7 in, 3 out]
        n38 = call <vilib>:"WPI_CANTalonSRX_SetOutput.vi"("Output"=w80, "MotorControlDevRef"=w81) -> ()  [unwired: 7 in, 3 out]
        n39 = Negate(x=w83) -> (-x=w79:dbl)
        n40 = call <vilib>:"WPI_CANTalonSRX_SetOutput.vi"("Output"=w79, "MotorControlDevRef"=w85) -> ()  [unwired: 7 in, 3 out]
        n41 = call <vilib>:"WPI_CANTalonSRX_SetOutput.vi"("Output"=w79, "MotorControlDevRef"=w84) -> ()  [unwired: 7 in, 3 out]
      }
      frame True {
        n42 = feedback #1() -> (w93:bool)  [unwired: 1 in]
        n43 = feedback #2() -> (w97:cluster{dbl, dbl}[])
        n44 = feedback #3() -> (w95:cluster{dbl, dbl}[])
        n45 = case shown="False" w93 {
          tunnel: w107 -> [w108 w159]
          tunnel: w106 -> [w110 w157]
          tunnel: w105 -> [_ w151]
          tunnel: w104 -> [_ w150]
          tunnel: w103 -> [_ w145]
          tunnel: w102 -> [_ w144]
          tunnel: w101 -> [w109 w141]
          tunnel: w100 -> [w122 _]
          tunnel: w99 -> [w121 _]
          tunnel: [w118 w130] -> w96
          tunnel: [w117 w131] -> w98
          tunnel: w97 -> [_ w131]
          tunnel: w95 -> [_ w130]
          tunnel: [w112 w128] -> w94
          frame False {
            n46 = call <vilib>:"WPI_EncoderReset.vi"("EncoderDevRef"=w108) -> ()  [unwired: 9 in, 2 out]
            n47 = call <vilib>:"WPI_EncoderReset.vi"("EncoderDevRef"=w109) -> ()  [unwired: 9 in, 2 out]
            n48 = call <userlib>:"IMUOrientRead.vi"("I2CDevRef"=w110, "Gyro Reset"=TRUE) -> ()  [unwired: 7 in, 7 out]
            n49 = Wait on Notification(notifier=w121, timeout in ms (-1)=0) -> (notification=w117:cluster{dbl, dbl}[], timed out?=w116:bool)  [unwired: 2 in, 2 out]
            n50 = Wait on Notification(notifier=w122, timeout in ms (-1)=0) -> (notification=w118:cluster{dbl, dbl}[], timed out?=w115:bool)  [unwired: 2 in, 2 out]
            n51 = Not(x=w116) -> (.not. x?=w114:bool)
            n52 = Not(x=w115) -> (.not. x?=w113:bool)
            n53 = And(x=w114, y=w113) -> (x .and. y?=w112:bool)
          }
          frame True {
            n54 = call <vilib>:"PID Setpoint Profile.vi"("setpoint profile"=w131) -> ("profile complete?"=w158:bool, "setpoint"=w137:dbl)  [unwired: 5 in, 2 out]
            n55 = call <vilib>:"WPI_EncoderGet.vi"("EncoderDevRef"=w159) -> ("Distance"=w143:dbl)  [unwired: 5 in, 5 out]
            n56 = call <vilib>:"PID Setpoint Profile.vi"("setpoint profile"=w130) -> ("profile complete?"=w161:bool, "setpoint"=w139:dbl)  [unwired: 5 in, 2 out]
            n57 = call <userlib>:"IMUOrientRead.vi"("I2CDevRef"=w157) -> ("Orient Y/R/P"=w156:T14)  [unwired: 8 in, 6 out]
            n58 = call <vilib>:"WPI_EncoderGet.vi"("EncoderDevRef"=w141) -> ("Distance"=w127:dbl)  [unwired: 5 in, 5 out]
            n59 = Wait (ms)(milliseconds to wait=u32 10) -> ()  [unwired: 1 out]
            n60 = Unbundle By Name(w156) -> ("Yaw Wind"=w155:dbl)
            n61 = And(x=w158, y=w161) -> ()  [unwired: 1 out]
            n62 = Negate(x=w143) -> (-x=w124:dbl)
            n63 = Add(x=w124, y=w127) -> (x+y=w126:dbl)
            n64 = Divide(x=w126, y=2.0) -> (x/y=w123:dbl)
            n65 = expression code="(x/180.0)*pi" "degrees to radians"(w155) -> (w140:dbl)
            n66 = call-poly <vilib>:"PID.vi"("output range"="Speed Range", "PID gains"="PID Speed gains", "process variable"=w123, "setpoint"=w137) -> ("output"=w154:dbl)  [unwired: 6 in, 1 out]
            n67 = Bundle(w123, "setpoint"=w137) -> (→"Waveform Chart":cluster{dbl, "setpoint":dbl})  [unwired: 1 in]
            n68 = call-poly <vilib>:"PID.vi"("output range"="Steer Range", "PID gains"="PID Steer gains", "process variable"=w140, "setpoint"=w139) -> ("output"=w153:dbl)  [unwired: 6 in, 1 out]
            "steer" <- w153
            n69 = Bundle("Yaw Wind"=w140, "setpoint"=w139) -> (→"Waveform Chart 2":cluster{"Yaw Wind":dbl, "setpoint":dbl})  [unwired: 1 in]
            n70 = Negate(x=w154) -> (-x=w142:dbl)
            "throttle" <- w142
            n71 = call <userlib>:"hmi_cheesy_drive.vi"("Quick Turn"=TRUE, "Wheel"=w153, "Throttle"=w142) -> ("Drive Data"=w152:cluster{"Left":dbl, "Right":dbl})  [unwired: 8 in]
            n72 = Unbundle By Name(w152) -> ("Left"=w148:dbl, "Right"=w149:dbl)
            n73 = Not(x="Finished PID") -> (.not. x?=w128:bool)
            n74 = call <vilib>:"WPI_CANTalonSRX_SetOutput.vi"("Output"=w148, "MotorControlDevRef"=w151) -> ()  [unwired: 7 in, 3 out]
            n75 = call <vilib>:"WPI_CANTalonSRX_SetOutput.vi"("Output"=w148, "MotorControlDevRef"=w150) -> ()  [unwired: 7 in, 3 out]
            n76 = Negate(x=w149) -> (-x=w146:dbl)
            n77 = call <vilib>:"WPI_CANTalonSRX_SetOutput.vi"("Output"=w146, "MotorControlDevRef"=w145) -> ()  [unwired: 7 in, 3 out]
            n78 = call <vilib>:"WPI_CANTalonSRX_SetOutput.vi"("Output"=w146, "MotorControlDevRef"=w144) -> ()  [unwired: 7 in, 3 out]
          }
        }
        n79 = feedback-in #1(w94) -> ()
        n80 = feedback-in #2(w98) -> ()
        n81 = feedback-in #3(w96) -> ()
      }
    }
  }
